vi "GetAvPowerN1911wHandle.vi"(6 "error in (no error)":errorcluster, 7 "NreadingsFromPwrMeter":i32=20 min=1 max=1000 step=1, 8 "IntervalBetweenReadings (mS)":i32=10 min=1 max=1000 step=1) -> (0 "Error out":errorcluster, 1 "VI dBSSD Power (dB)":dbl format="%#.10f", 2 "Computed LinMean Power (dBm)":dbl format="%#.10f", 3 "VI dBMean Power (dBm)":dbl format="%#.10f", 9 "VI dBRange Power reading (dB)":dbl format="%#.10f", 10 "VI dBMin Power reading (dBm)":dbl format="%#.10f", 11 "VI dBMax Power reading (dBm)":dbl format="%#.10f")   [LabVIEW 2009]
doc: "Reads the power from the N1911A power meter."
uses:
  <vilib>/Analysis/baseanly.llb/Multimode.vi
  <vilib>/Analysis/NI_AALBase.lvlib
panel:
  in  "ModeIntervals":i32 min=0 max=1000 step=1
  out "dBPwrMode3 (dBm)":dbl format="%#.10f"
  out "dBPwrMode2 (dBm)":dbl format="%#.10f"
  out "dBPwrMode1 (dBm)":dbl format="%#.10f"
  out "PwrAveragingLoopCount":i32
  in  "HistogramIntervals":i32=50 min=1 max=1000 step=1
  out "dB Readings Histogram":T1(graph)
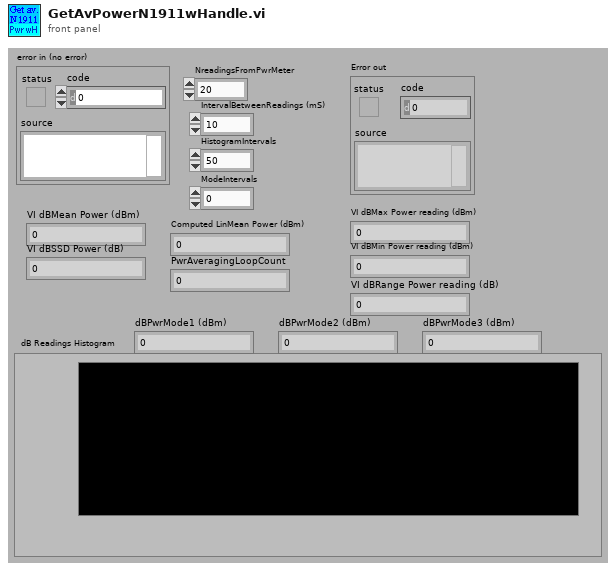
[diagram p1: front panel]
types:
  T1 = cluster{"X Values":dbl[], "Histogram: h(x)":i32[]}
  T2 = cluster{"Modes[0]":dbl, "Modes[1]":dbl, "Modes[2]":dbl}
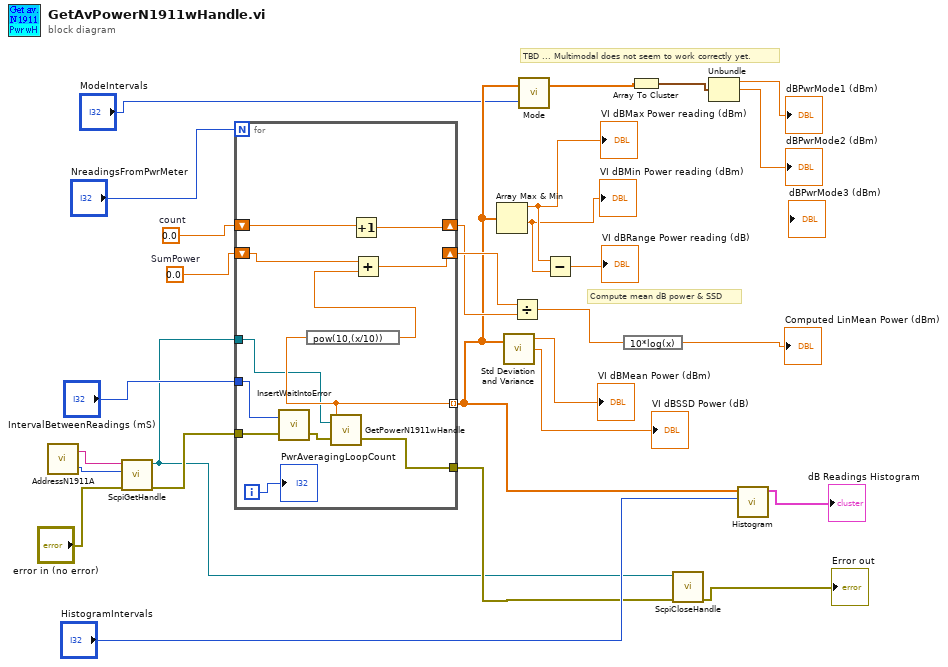
[diagram p0: block diagram]
diagram:
  w25 = 0.0  # count
  w28 = 0.0  # SumPower
  # "TBD ... Multimodal does not seem to work correctly yet."
  # "Compute mean dB power & SSD"
  n1 = call "AddressN1911A.vi"() -> ("Port"=w4:i32, "IP address"=w5:string)  [unwired: 2 in]
  n2 = call "ScpiGetHandle.vi"("error in (no error)"="error in (no error)", "TCP port"=w4, "IP Address"=w5) -> ("Error out"=w6:errorcluster, "connection ID"=w1:refnum<k5>)  [unwired: 6 in]
  n3 = for {
    N: "NreadingsFromPwrMeter" -> [_]
    shift-right: [w39] -> w27
    shift-left: w28 -> [w40]
    tunnel: [w38] -> w2
    shift-right: [w36] -> w24
    shift-left: w25 -> [w37]
    tunnel: [w33] -> w14 mode=indexing
    tunnel: "IntervalBetweenReadings (mS)" -> [w34]
    tunnel: w1 -> [w30]
    tunnel: w6 -> [w29]
    i -> [w31]
    n4 = call "InsertWaitIntoError.vi"("error in (no error)"=w29, "Wait (msecs)"=w34) -> ("error out"=w35:errorcluster)  [unwired: 1 in]
    n5 = call "GetPowerN1911wHandle.vi"("error in (no error)"=w35, "connection ID"=w30) -> ("Error out"=w38:errorcluster, "Power returned (dBm)"=w33:dbl)
    n6 = expression code="pow(10,(x/10))"(w33) -> (w32:dbl)
    n7 = Increment(x=w37) -> (x+1=w36:dbl)
    n8 = Add(x=w40, y=w32) -> (x+y=w39:dbl)
    "PwrAveragingLoopCount" <- w31
  }
  n9 = Array Max & Min(array=w14) -> (max value=w21:dbl, min value=w20:dbl)  [unwired: 2 out]
  "VI dBMax Power reading (dBm)" <- w21
  "VI dBMin Power reading (dBm)" <- w20
  n10 = call <vilib>:"Std Deviation and Variance.vi"("X"=w14) -> ("mean"=→"VI dBMean Power (dBm)":dbl, "standard deviation"=→"VI dBSSD Power (dB)":dbl)  [unwired: 1 in, 1 out]
  n11 = Divide(x=w27, y=w24) -> (x/y=w17:dbl)
  n12 = call-poly <vilib>:"Mode.vi"("intervals"="ModeIntervals", "X"=w14) -> ("Modes"=w13:dbl[])  [unwired: 1 out]
  n13 = Subtract(x=w21, y=w20) -> (x-y=→"VI dBRange Power reading (dB)":dbl)
  n14 = expression code="10*log(x)"(w17) -> (→"Computed LinMean Power (dBm)":dbl)
  n15 = Array To Cluster(array=w13) -> (cluster=w12:T2)
  n16 = call "ScpiCloseHandle.vi"("error in (no error)"=w2, "connection ID"=w1) -> ("Error out"=→"Error out":errorcluster)  [unwired: 8 in]
  n17 = Unbundle(w12) -> ("Modes[0]"=→"dBPwrMode1 (dBm)":dbl, "Modes[1]"=→"dBPwrMode2 (dBm)":dbl)  [unwired: 1 out]
  n18 = call <vilib>:"Histogram.vi"("intervals"="HistogramIntervals", "X"=w14) -> ("Histogram Graph"=→"dB Readings Histogram":T1)  [unwired: 6 in, 3 out]
